vi "RDV-sortData.vi"(8 "error in (no error)":errorcluster, 11 "RDV-Reflection_Data_viewer in":refnum<class "RDV-Reflection_Data_viewer.lvclass">) -> (0 "error out":errorcluster, 3 "RDV-Reflection_Data_viewer out":refnum<class "RDV-Reflection_Data_viewer.lvclass">)   [LabVIEW 2020, in "RDV-Reflection_Data_viewer.lvclass"]
uses:
  RDV-Reflection_Data_viewer.lvclass
  RDV-Reflection_Data_viewer.lvclass/RDV-Reflection_Data_viewer.ctl
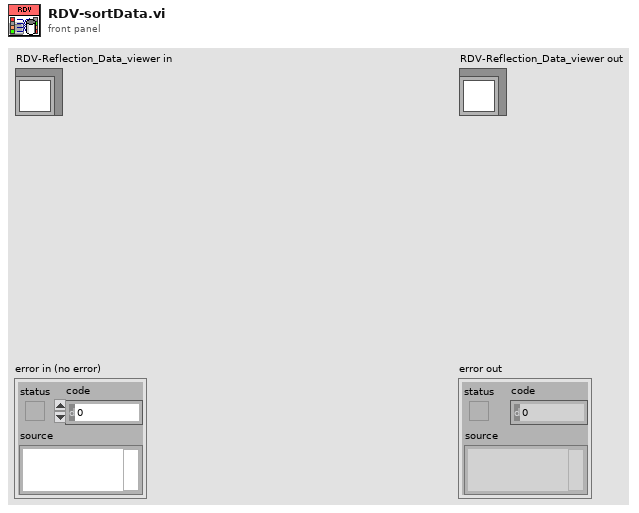
[diagram p1: front panel]
types:
  T1 = typedef "RDV-Reflection_Data_viewer.lvclass/RDV-DATA_MAP.ctl" = map{string, cluster{"filename without extension":string, "Common Format":T2}}
  T2 = typedef "RFH-Reflection_File_Handler.lvlib/RFH-common_data_format.ctl" = cluster{"Frequency":dbl[], "Reflection'":dbl[], "Reflection''":dbl[], "Permativity'":dbl[], "Permativity''":dbl[]}
  T3 = cluster{"filename without extension":string, "Common Format":T2}
  T4 = cluster{"Frequency":dbl[], "Permativity''":dbl[]}
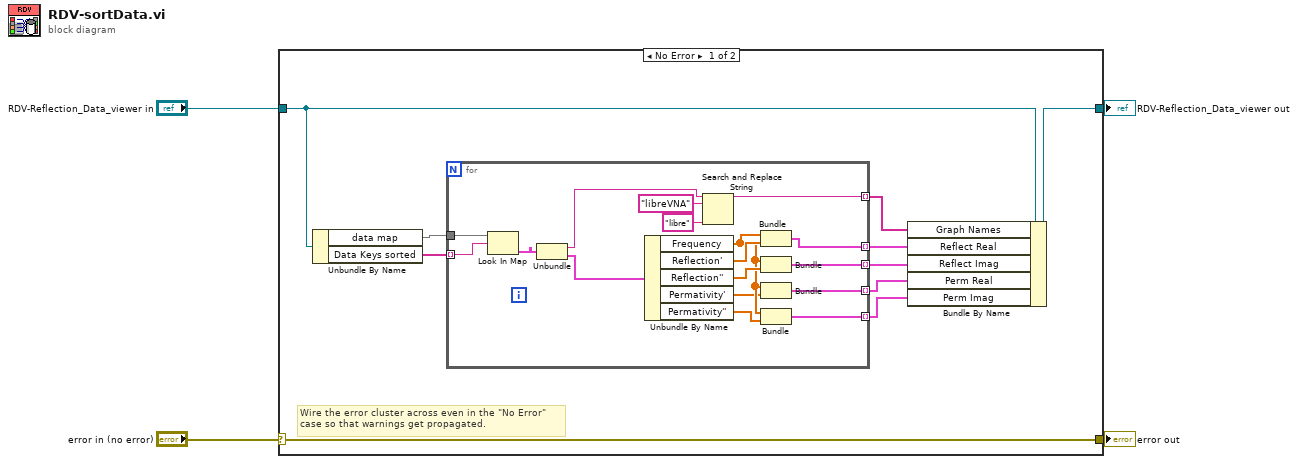
[diagram p0: block diagram]
diagram:
  n1 = case shown="No Error" "error in (no error)" {
    selector: "error in (no error)" -> [w14 w33]
    tunnel: [w14 w33] -> w3
    tunnel: [w10 w32] -> w1
    tunnel: "RDV-Reflection_Data_viewer in" -> [w13 w32]
    frame No Error {
      # "Wire the error cluster across even in the \"No Error\"\ncase so that warnings get propagated."
      n2 = Unbundle By Name(w13) -> ("data map"=w12:T1, "Data Keys sorted"=w11:string[])
      n3 = for {
        tunnel: [w29] -> w8 mode=indexing
        tunnel: [w28] -> w7 mode=indexing
        tunnel: w12 -> [w23]
        tunnel: w11 -> [w22] mode=indexing
        tunnel: [w20] -> w9 mode=indexing
        tunnel: [w16] -> w6 mode=indexing
        tunnel: [w15] -> w5 mode=indexing
        n4 = Look In Map(map=w23, key=w22) -> (value=w21:T3)  [unwired: 1 in, 1 out]
        n5 = Unbundle(w21) -> ("filename without extension"=w25:string, "Common Format"=w24:T2)
        n6 = Unbundle By Name(w24) -> ("Frequency"=w19:dbl[], "Reflection'"=w31:dbl[], "Reflection''"=w30:dbl[], "Permativity'"=w18:dbl[], "Permativity''"=w17:dbl[])
        n7 = Search and Replace String(input string=w25, search string="libreVNA", replace string="libre" ("replace string (\"\")")) -> (result string=w20:string)  [unwired: 5 in, 3 out]
        n8 = Bundle("Frequency"=w19, "Reflection'"=w31) -> (w29:cluster{"Frequency":dbl[], "Reflection'":dbl[]})  [unwired: 1 in]
        n9 = Bundle("Frequency"=w19, "Reflection''"=w30) -> (w28:cluster{"Frequency":dbl[], "Reflection''":dbl[]})  [unwired: 1 in]
        n10 = Bundle("Frequency"=w19, "Permativity'"=w18) -> (w16:cluster{"Frequency":dbl[], "Permativity'":dbl[]})  [unwired: 1 in]
        n11 = Bundle("Frequency"=w19, "Permativity''"=w17) -> (w15:T4)  [unwired: 1 in]
      }
      n12 = Bundle By Name(cluster=w13, "Graph Names"=w9, "Reflect Real"=w8, "Reflect Imag"=w7, "Perm Real"=w6, "Perm Imag"=w5) -> (w10:refnum<class "RDV-Reflection_Data_viewer.lvclass">)
    }
    frame Error {
    }
  }
  "error out" <- w3
  "RDV-Reflection_Data_viewer out" <- w1
